vi "Convert to percentage.vi"(11 "Value":sgl) -> (3 "%":sgl)   [LabVIEW 2015, in "Utility.lvlib"]
uses:
  Utility.lvlib
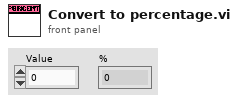
[diagram p1: front panel]
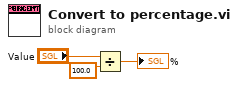
[diagram p0: block diagram]
diagram:
  n1 = Divide(x="Value", y=sgl 100.0) -> (x/y=→"%":sgl)
